vi "IMAQ_SUM.vi"(11 "Image":T1) -> (2 "Sum":sgl, 3 "Image 2":T1)   [LabVIEW 2011]
uses:
  IMAQ Image.ctl
  NI_Vision_Development_Module.lvlib
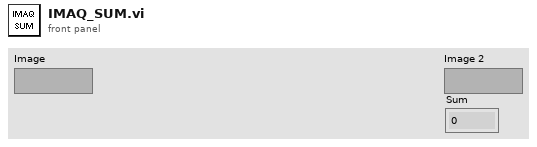
[diagram p1: front panel]
types:
  T1 = typedef "IMAQ Image.ctl" = refnum<image>
  T2 = cluster{"histogram":u32[], "Minimal Value":sgl, "Maximal Value":sgl, "Starting Value":sgl, "Interval Width":sgl, "Mean Value":sgl, "Standard  Variation":sgl, "Area (pixels)":i32}
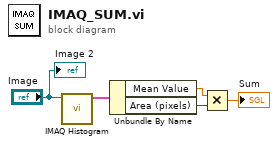
[diagram p0: block diagram]
diagram:
  n1 = call "IMAQ Histogram"("Image"="Image") -> ("Histogram Report"=w5:T2)  [unwired: 9 in, 1 out]
  n2 = Unbundle By Name(w5) -> ("Mean Value"=w4:sgl, "Area (pixels)"=w3:i32)
  n3 = Multiply(x=w4, y=w3) -> (x*y=→"Sum":sgl)
  "Image 2" <- "Image"
